vi "Dbl Array_Place Line between points.vi"(7 "Digital":bool, 9 "Second Index":i32, 10 "First Index":i32, 11 "Dbl Array":dbl[](array[numeric])) -> (3 "Dbl Array Out":dbl[](array[numeric]))   [LabVIEW 2024]
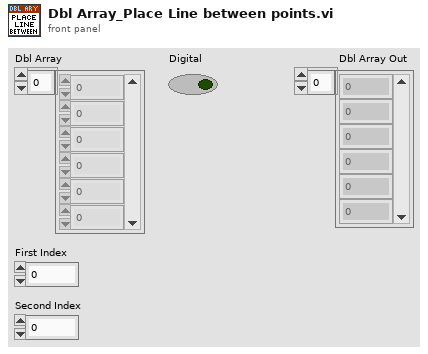
[diagram p1: front panel]
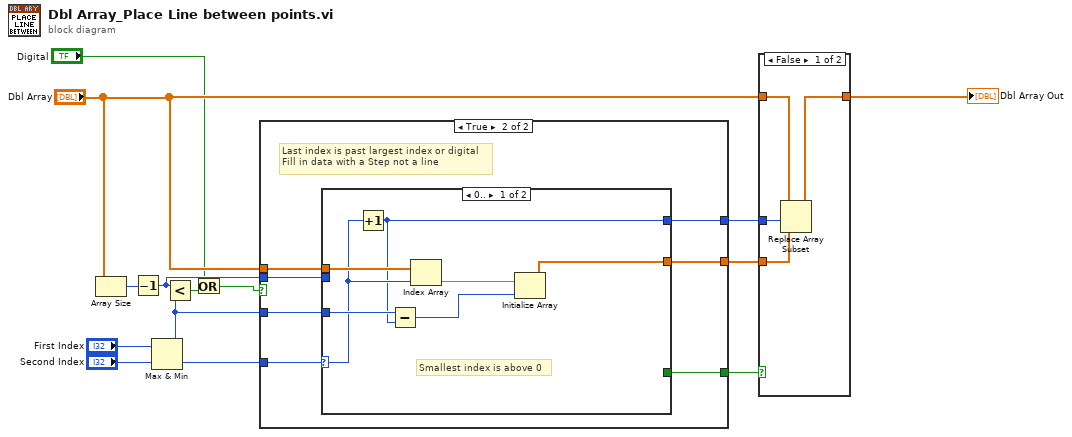
[diagram p0: block diagram]
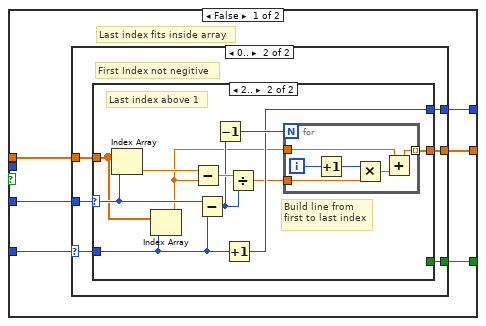
[diagram p2: hidden frame]
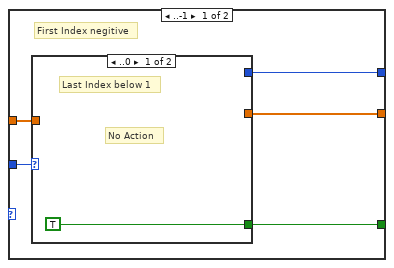
[diagram p3: hidden frame]
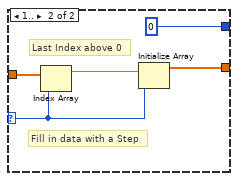
[diagram p4: hidden frame]
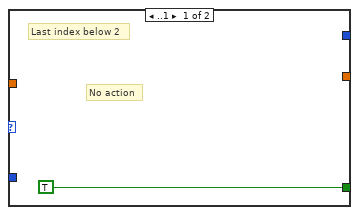
[diagram p5: hidden frame]
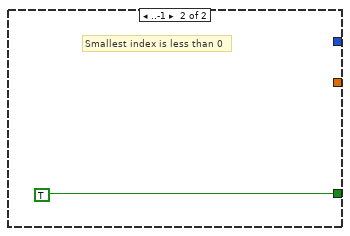
[diagram p6: hidden frame]
diagram:
  n1 = Array Size(array="Dbl Array") -> (size(s)=w6:i32)
  n2 = Decrement(x=w6) -> (x-1=w3:i32)
  n3 = Max & Min(x="First Index", y="Second Index") -> (max(x,y)=w5:i32, min(x,y)=w12:i32)
  n4 = Less?(x=w3, y=w5) -> (x < y?=w4:bool)
  n5 = Or(x="Digital", y=w4) -> (x .or. y?=w2:bool)
  n6 = case shown="True" w2 {
    tunnel: w12 -> [w20 w62]
    tunnel: [w19 w57] -> w10
    tunnel: [w18 w60] -> w9
    tunnel: [w17 w61] -> w8
    tunnel: "Dbl Array" -> [w16 w59]
    tunnel: w5 -> [w15 w56]
    tunnel: w3 -> [_ w58]
    frame False {
      # "Last index fits inside array"
      n7 = case shown="0.." w20 {
        selector: w20 -> [_ w32]
        tunnel: w15 -> [w25 w37]
        tunnel: w16 -> [w24 w36]
        tunnel: [w23 w35] -> w19
        tunnel: [w22 w34] -> w18
        tunnel: [w21 w33] -> w17
        frame ..-1 {
          # "First Index negitive"
          n8 = case shown="..0" w25 {
            selector: w25 -> [_ w30]
            tunnel: w24 -> [_ w31]
            tunnel: [_ w28] -> w23
            tunnel: [_ 0] -> w22
            tunnel: [TRUE _] -> w21
            frame ..0 {
              # "No Action"
              # "Last Index below 1"
            }
            frame 1.. {
              # "Fill in data with a Step"
              # "Last Index above 0"
              n9 = Index Array(array=w31, index=w30) -> (element=w29:dbl)
              n10 = Initialize Array(w29, w30) -> (w28:dbl[])
            }
          }
        }
        frame 0.. {
          # "First Index not negitive"
          n11 = case shown="2.." w37 {
            selector: w37 -> [_ w48]
            tunnel: w36 -> [_ w44]
            tunnel: [_ w39] -> w35
            tunnel: [_ w42] -> w34
            tunnel: [TRUE _] -> w33
            tunnel: w32 -> [_ w43]
            frame ..1 {
              # "No action"
              # "Last index below 2"
            }
            frame 2.. {
              # "Last index above 1"
              # "Build line from\nfirst to last index"
              n12 = Index Array(array=w44, index=w48) -> (element=w49:dbl)
              n13 = Index Array(array=w44, index=w43) -> (element=w40:dbl)
              n14 = Subtract(x=w49, y=w40) -> (x-y=w47:dbl)
              n15 = Subtract(x=w48, y=w43) -> (x-y=w46:i32)
              n16 = Decrement(x=w46) -> (x-1=w45:i32)
              n17 = Increment(x=w43) -> (x+1=w42:i32)
              n18 = Divide(x=w47, y=w46) -> (x/y=w41:dbl)
              n19 = for {
                N: w45 -> [_]
                tunnel: w41 -> [w53]
                tunnel: w40 -> [w51]
                tunnel: [w50] -> w39 mode=indexing
                i -> [w55]
                n20 = Increment(x=w55) -> (x+1=w54:i32)
                n21 = Multiply(x=w54, y=w53) -> (x*y=w52:dbl)
                n22 = Add(x=w51, y=w52) -> (x+y=w50:dbl)
              }
            }
          }
        }
      }
    }
    frame True {
      # "Last index is past largest index or digital\nFill in data with a Step not a line"
      n23 = case shown="0.." w62 {
        selector: w62 -> [w65 _]
        tunnel: [_ TRUE] -> w61
        tunnel: [w63 _] -> w60
        tunnel: w59 -> [w69 _]
        tunnel: w58 -> [_ _]
        tunnel: [w67 _] -> w57
        tunnel: w56 -> [w66 _]
        frame 0.. {
          # "Smallest index is above 0"
          n24 = Increment(x=w65) -> (x+1=w63:i32)
          n25 = Subtract(x=w66, y=w63) -> (x-y=w64:i32)
          n26 = Index Array(array=w69, index=w65) -> (element=w68:dbl)
          n27 = Initialize Array(w68, w64) -> (w67:dbl[])
        }
        frame ..-1 {
          # "Smallest index is less than 0"
        }
      }
    }
  }
  n28 = case shown="False" w8 {
    tunnel: "Dbl Array" -> [w74 w75]
    tunnel: [w73 w75] -> w11
    tunnel: w10 -> [w72 _]
    tunnel: w9 -> [w71 _]
    frame False {
      n29 = Replace Array Subset(array=w74, new element=w72, index=w71) -> (w73:dbl[])
    }
    frame True {
    }
  }
  "Dbl Array Out" <- w11
